vi "Resolve Variant Example.vi"() -> ()   [LabVIEW 2020, in "Futures-Examples.lvlib"]
uses:
  Futures-Examples.lvlib
  Promises/Promise/Promise.lvclass/Promise.ctl
  Promises/Future/Future.lvclass/Future.ctl
  Promises/Variant/Variant.lvclass/Variant.ctl
  1a02a226-e3b3-4612-8974-3f7179bfb47d.vi
  Promises/Variant/Read.vi
  Promises/Future/Wait.vi
  Promises/Future/Future.lvclass
  Promises/Variant/Variant.lvclass
  Promises/Promise/Promise.lvclass
panel:
  out "error out":errorcluster
  out "Result":string
  in  "Value":dbl
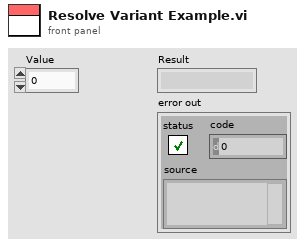
[diagram p1: front panel]
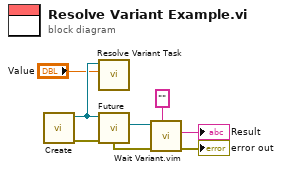
[diagram p0: block diagram]
diagram:
  n1 = call "Create.vi"() -> ("error out"=w2:errorcluster, "Promise"=w7:refnum<class "Promise.lvclass">)  [unwired: 10 in]
  n2 = call "Resolve Variant Task.vi"("Value"="Value", "Promise"=w7) -> ()  [unwired: 10 in]
  n3 = call "Future.vi"("Promise in"=w7) -> ("Future"=w6:refnum<class "Future.lvclass">)  [unwired: 9 in, 1 out]
  n4 = call "Wait Variant.vim"("Result Type (Variant)"="", "error in (no error)"=w2, "Future in"=w6) -> ("error out"=→"error out":errorcluster, "Result"=→"Result":string)  [unwired: 7 in]
